vi "SPI Engine 64-bit.vi"(8 "error in":errorcluster, 10 "SPI Read Data":T4, 11 "SPI Engine Resources":T1={"To SPI Engine Data FIFO"="DLU To SPI Engine Data FIFO", "From SPI Engine Data FIFO"="SPI Engine to DLU Data FIFO", "Data to SPI Engine Cache Register"="Data to SPI Engine (Cache)", "SPI Transaction Settings Cache Register"="SPI PHY Settings to SPI Engine (Cache)"}) -> (0 "error out":errorcluster, 1 "Chip Select":u8, 2 "SPI Write Data":T5, 3 "SPI Engine Resources":T1={"To SPI Engine Data FIFO"="DLU To SPI Engine Data FIFO", "From SPI Engine Data FIFO"="SPI Engine to DLU Data FIFO", "Data to SPI Engine Cache Register"="Data to SPI Engine (Cache)", "SPI Transaction Settings Cache Register"="SPI PHY Settings to SPI Engine (Cache)"})   [LabVIEW 2015, in "SPI API.lvlib"]
doc: "This VI is the top level VI of the SPI Engine, and acts as a wrapper for the Engine Core and the VIs that supply commands to the Engine Core and return the responses read from the SPI bus. The SPI Engine directly handles the communication on the SPI bus according to the commands that are queued to it."
uses:
  SPI API.lvlib
  <userlib>/_NI SPI IP/FPGA/Controllers/Public/Spi Master Outputs.ctl
  <userlib>/_NI SPI IP/FPGA/Controllers/Public/Spi Master Inputs.ctl
  Controls/SPI API Response Data 64-bit.ctl
  Controls/SPI API Data 64-bit.ctl
  Controls/SPI Engine Resources 64-bit.ctl
  Get SPI Engine Commands 64-bit.vi
  SPI Engine Core 64-bit.vi
  Send SPI Engine Response 64-bit.vi
  <userlib>/_NI SPI IP/FPGA/Controllers/NI SPI IP FPGA.lvlib
panel:
  out "Output Data":T2
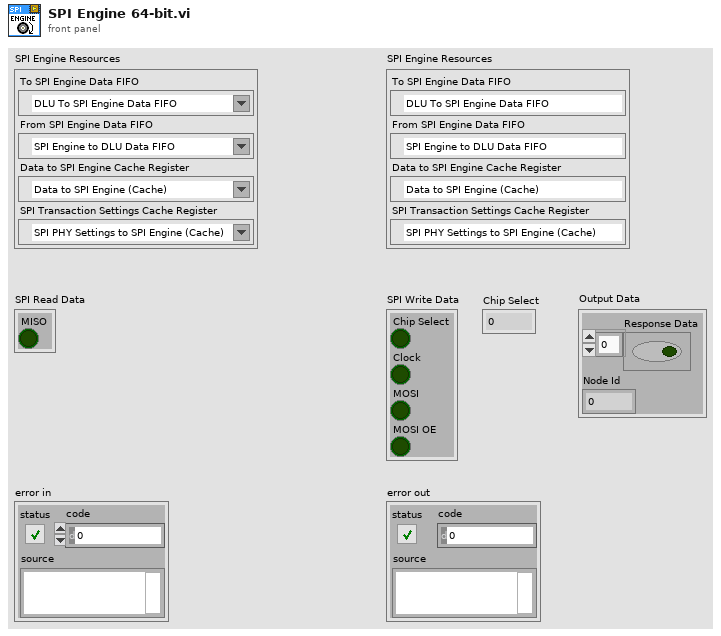
[diagram p1: front panel]
types:
  T1 = typedef "SPI API.lvlib/SPI Engine Resources 64-bit.ctl" = cluster{"To SPI Engine Data FIFO":refnum<k21>, "From SPI Engine Data FIFO":refnum<k21>, "Data to SPI Engine Cache Register":refnum<k21>, "SPI Transaction Settings Cache Register":refnum<k21>}
  T2 = typedef "SPI API.lvlib/SPI API Response Data 64-bit.ctl" = cluster{"Response Data":T3, "Node Id":u16}
  T3 = typedef "SPI API.lvlib/SPI API Data 64-bit.ctl" = bool[]
  T4 = typedef "NI SPI IP FPGA.lvlib/Spi Master Inputs.ctl" = cluster{"MISO":bool}
  T5 = typedef "NI SPI IP FPGA.lvlib/Spi Master Outputs.ctl" = cluster{"Chip Select":bool, "Clock":bool, "MOSI":bool, "MOSI OE":bool}
  T6 = typedef "SPI API.lvlib/SPI API Transaction Packet 64-bit.ctl" = cluster{"Start Strobe":bool, "SPI Data":T3, "SPI Settings":T7}
  T7 = typedef "SPI API.lvlib/SPI Transaction Settings.ctl" = cluster{"Chip Select ID":u8, "SPI Physical Settings":T8}
  T8 = typedef "NI SPI IP FPGA.lvlib/Transfer Settings.ctl" = cluster{"Divide Value":u8, "Transfer Length (bits)":u8, "CS Asserted Polarity":bool, "Clock Polarity (CPOL)":bool, "Clock Phase (CPHA)":bool, "Lengthen MISO Setup":bool, "Direction Change Bit":u8, "MOSI Starts as Output":bool, "Tristatable MOSI":bool}
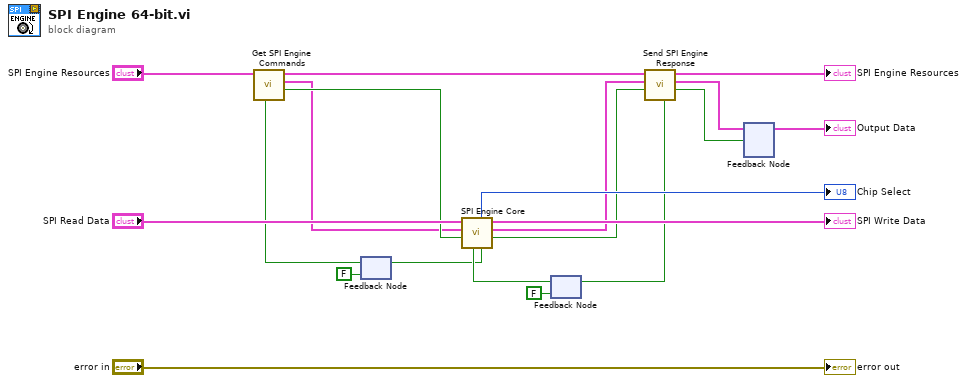
[diagram p0: block diagram]
diagram:
  n1 = feedback #1(FALSE ("ready for input")) -> (w11:bool)
  n2 = call-poly "Get SPI Engine Commands.vi"("Ready for Output"=w11, "SPI Engine Resources"="SPI Engine Resources") -> ("Output Valid"=w10:bool, "SPI Transaction Packet"=w1:T6, "SPI Engine Resources"=w8:T1)  [unwired: 5 in, 2 out]
  n3 = feedback #2(FALSE ("Ready for Input")) -> (w16:bool)
  n4 = call-poly "SPI Engine Core.vi"("Ready for Output"=w16, "Input Valid"=w10, "SPI Transaction Packet"=w1, "SPI DIO Input"="SPI Read Data") -> ("Output Valid"=w4:bool, "SPI Output Data"=w3:T2, "SPI DIO Output"=→"SPI Write Data":T5, "Ready For Input"=w2:bool, "Chip Select ID"=→"Chip Select":u8)  [unwired: 3 in]
  n5 = feedback-in #1(w2) -> ()
  n6 = call-poly "Send SPI Engine Response.vi"("Input Valid"=w4, "Response Data"=w3, "SPI Engine Resources"=w8) -> ("New Data Sent?"=w5:bool, "Output Data"=w6:T2, "SPI Engine Resources"=→"SPI Engine Resources":T1, "Ready for Input"=w9:bool)  [unwired: 4 in, 1 out]
  n7 = feedback-in #2(w9) -> ()
  n8 = feedback-in #3(w6, w5) -> ()
  n9 = feedback #3() -> (→"Output Data":T2)  [unwired: 1 in]
  "error out" <- "error in"
